vi "Reverse_Message_Hex_String.vi"(0 "Input String":string="00 FF 00 FF", 11 "Error In":errorcluster) -> (4 "Output String":string, 15 "Error Out":errorcluster)   [LabVIEW 2014]
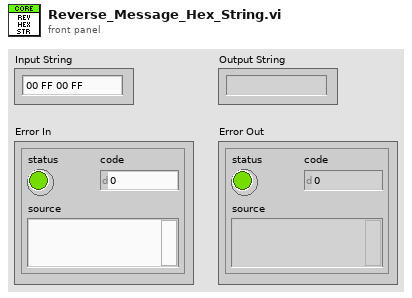
[diagram p1: front panel]
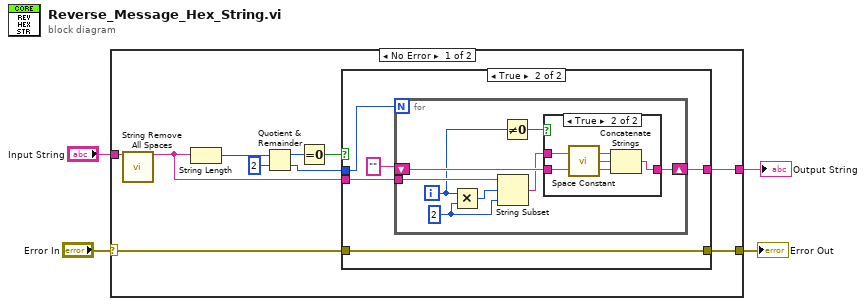
[diagram p0: block diagram]
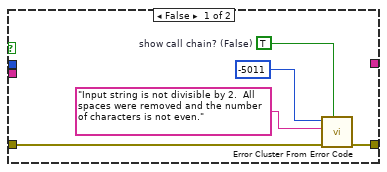
[diagram p2: hidden frame]
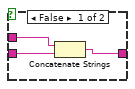
[diagram p3: hidden frame]
diagram:
  n1 = case shown="No Error" "Error In" {
    selector: "Error In" -> [w5 w40]
    tunnel: "Input String" -> [w14 _]
    tunnel: [w7 _] -> w3
    tunnel: [w6 w40] -> w1
    frame No Error {
      n2 = call "String Remove All Spaces.vi"("Input String"=w14) -> ("Spaces Removed"=w13:string)  [unwired: 13 in, 1 out]
      n3 = String Length(string=w13) -> (length=w12:i32)
      n4 = Quotient & Remainder(x=w12, y=2) -> (x-y*floor(x/y)=w10:i32, floor(x/y)=w8:i32)
      n5 = Equal To 0?(x=w10) -> (x = 0?=w9:bool)
      n6 = case shown="True" w9 {
        tunnel: w13 -> [_ w23]
        tunnel: w8 -> [_ w22]
        tunnel: [_ w21] -> w7
        tunnel: [w19 w20] -> w6
        tunnel: w5 -> [w18 w20]
        frame False {
          w15 = TRUE  # show call chain? (False)
          n7 = call <vilib>:"Error Cluster From Error Code.vi"("show call chain? (False)"=w15, "error in (no error)"=w18, "error message (\"\")"="Input string is not divisible by 2.  All spaces were removed and the number of characters is not even.", "error code (0)"=-5011) -> ("error out"=w19:errorcluster)  [unwired: 5 in]
        }
        frame True {
          n8 = for {
            N: w22 -> [_]
            shift-right: [w30] -> w21
            shift-left: "" -> [w31]
            tunnel: w23 -> [w32]
            i -> [w25]
            w29 = 2 ("length (rest)")
            n9 = Multiply(x=w25, y=w29) -> (x*y=w28:i32)
            n10 = String Subset(string=w32, offset (0)=w28, length (rest)=w29) -> (substring=w27:string)
            n11 = Not Equal To 0?(x=w25) -> (x != 0?=w26:bool)
            n12 = case shown="True" w26 {
              tunnel: w31 -> [w35 w39]
              tunnel: [w33 w38] -> w30
              tunnel: w27 -> [w34 w37]
              frame False {
                n13 = Concatenate Strings(w34, w35) -> (w33:string)
              }
              frame True {
                n14 = call <vilib>:"Space Constant.vi"() -> ("String"=w36:string)
                n15 = Concatenate Strings(w37, w36, w39) -> (w38:string)
              }
            }
          }
        }
      }
    }
    frame Error {
    }
  }
  "Error Out" <- w1
  "Output String" <- w3
